vi "RT_Main.vi"() -> ()   [LabVIEW 2024]
uses:
  Type Definitions/FIFO_Health.ctl
  Type Definitions/FPGA_routine_pulsing_typedef.ctl
  <vilib>/Utility/error.llb/Error Cluster From Error Code.vi
  <vilib>/rvi/errors/niLvFpgaAdjustHostInterfaceError.vi
  <vilib>/RVI Host/nirviSupport.llb/nirviErrorClusterFromErrorCode.vi
  <vilib>/rvi/interface/nirviReadWriteControl/nirviReadWriteControl.xnode
  <vilib>/rvi/interface/nirviMethod/nirviMethod.xnode
  <vilib>/FPGAPlugInAG/Dynamic/niLvFpga_ReadFifo_Dynamic.vi
  <vilib>/rvi/errors/niLvFpgaMergeErrorWithErrorCode.vi
  NiFpgaLv.dll
  <vilib>/rvi/interface/Simulation/niFpgaSimulationCallBeginRW.vi
  <vilib>/rvi/interface/nirviMethod/StockFPGA_InlinedMethodWaitForMultipleIRQ.vi
  <vilib>/FPGAPlugInAG/Dynamic/niLvFpga_WaitOnIrq_Dynamic.vi
  <vilib>/FPGAPlugInAG/Dynamic/niLvFpga_AcknowledgeIrq_Dynamic.vi
  <vilib>/rvi/interface/nirviMethod/StockFPGA_InlinedMethodWaitForSingleIRQ.vi
panel:
  out "Data Streaming Start":bool
  out "Triggers Start":bool
  out "Packet Start":bool
  out "RT_FPGA_FIFO_health":T1
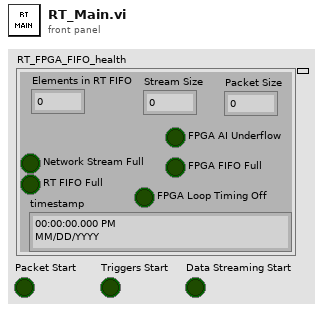
[diagram p1: front panel]
types:
  T1 = typedef "FIFO_Health.ctl" = cluster{"Elements in RT FIFO":i32, "Network Stream Full":bool, "RT FIFO Full":bool, "FPGA AI Underflow":bool, "FPGA FIFO Full":bool, "FPGA Loop Timing Off":bool, "timestamp":timestamp, "Stream Size":u32, "Packet Size":u32}
  T2 = cluster{"RT FIFO":refnum<k33>, "RT writer":refnum<k21>}
  T3 = typedef "FPGA_routine_pulsing_typedef.ctl" = cluster{"Pulsing":bool, "Pulse duration (uS)":u32, "Pulse Period (uS)":u32}
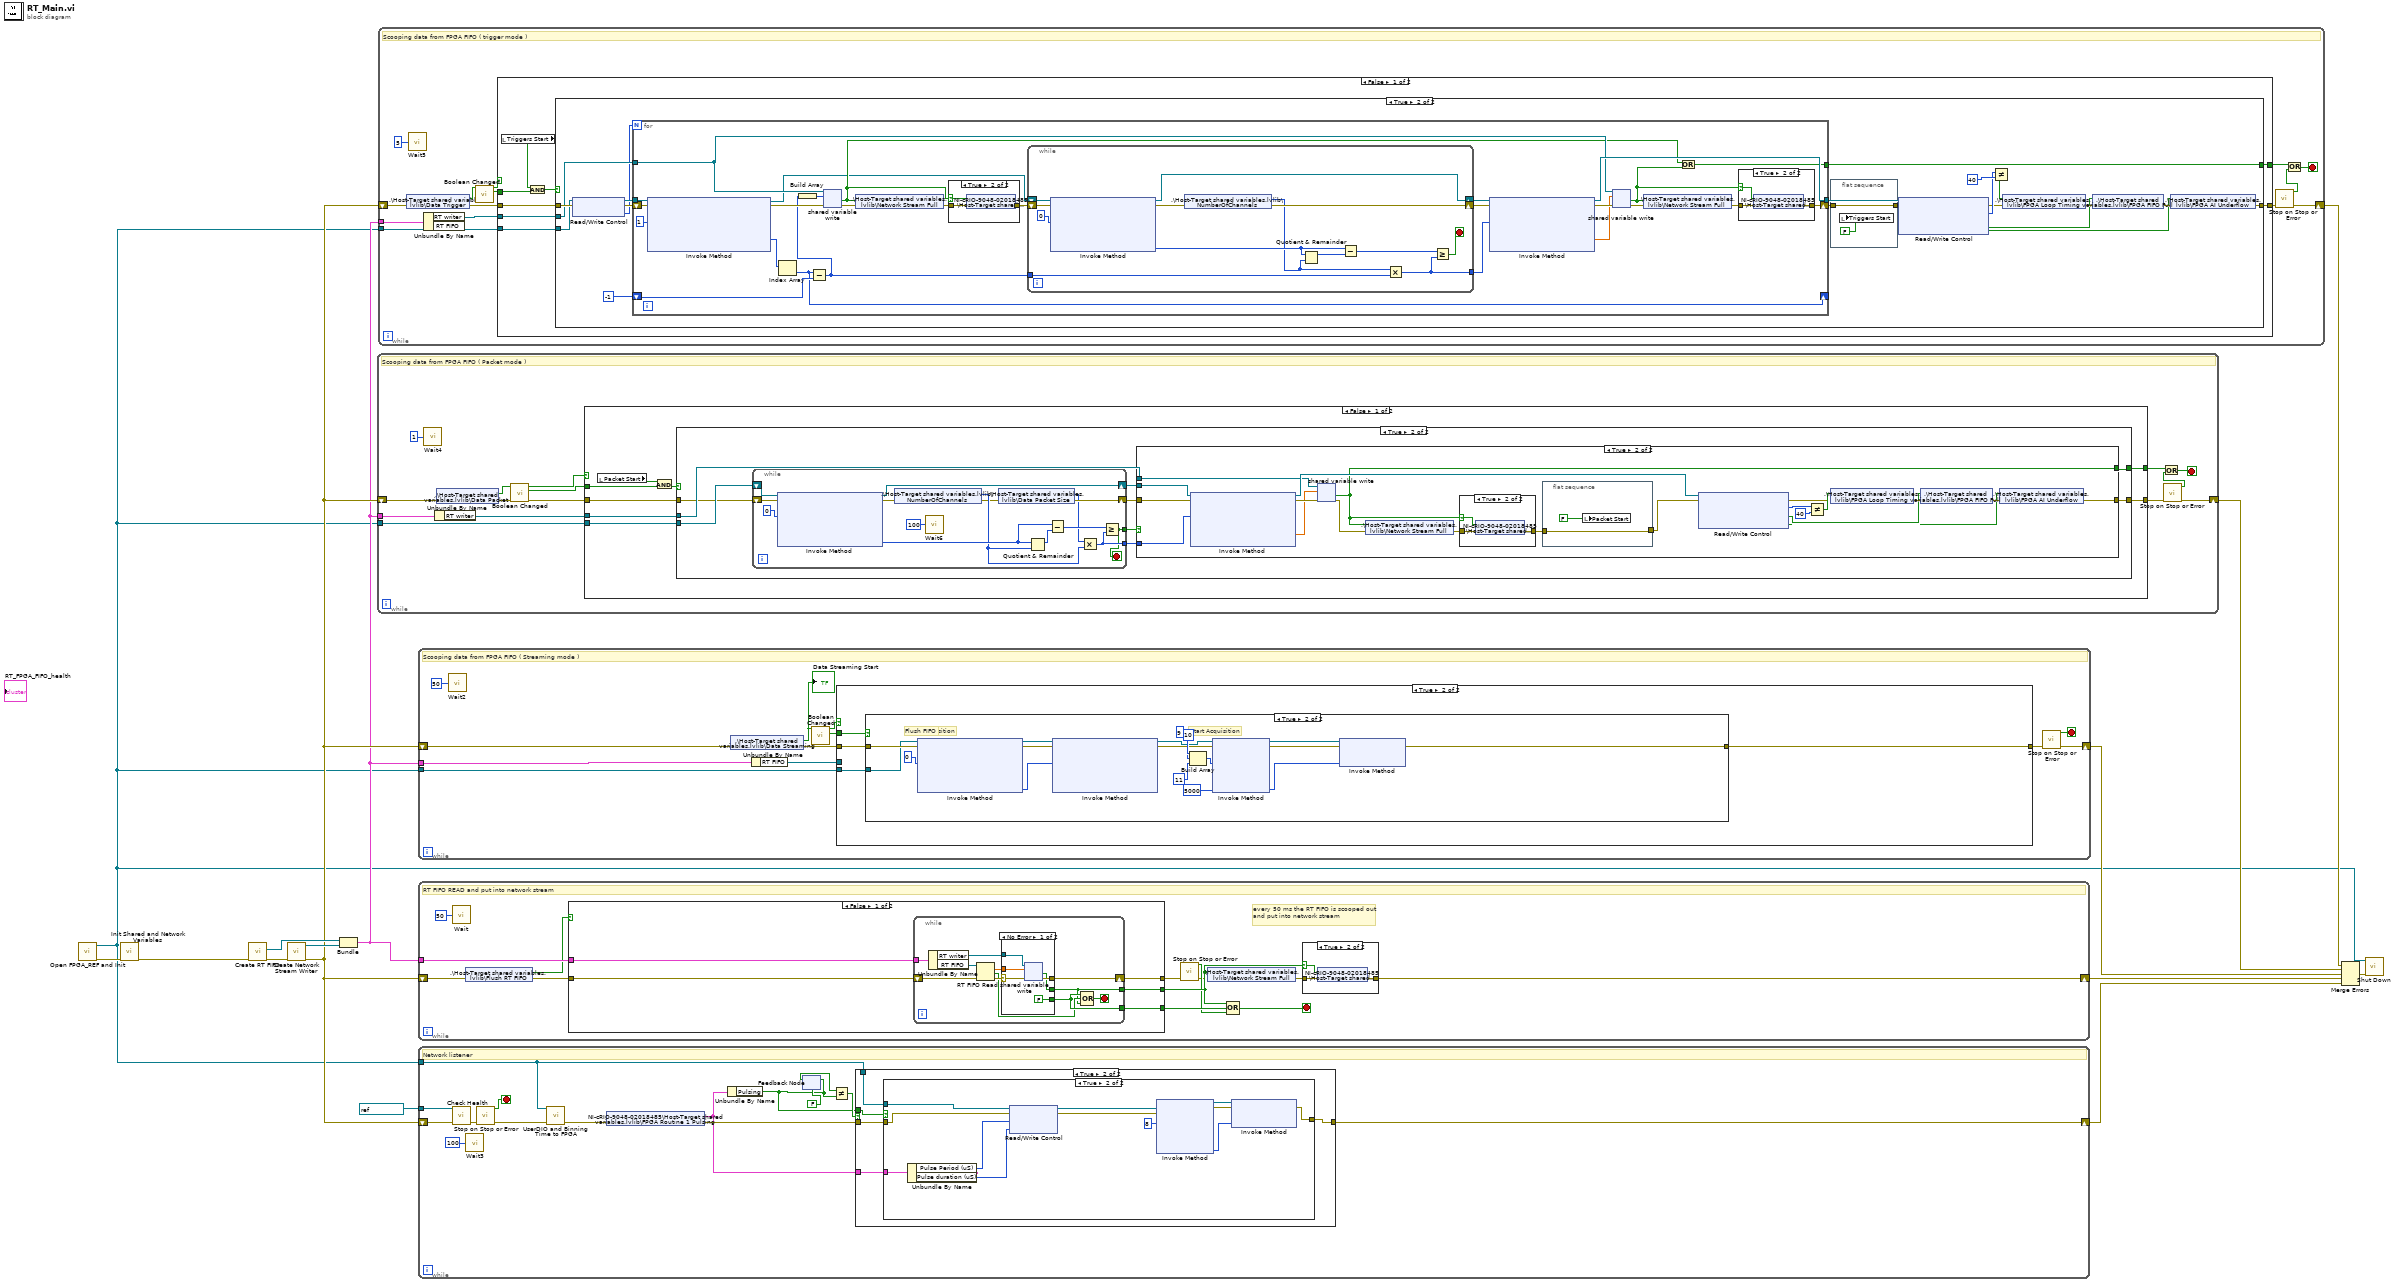
[diagram p0: block diagram]
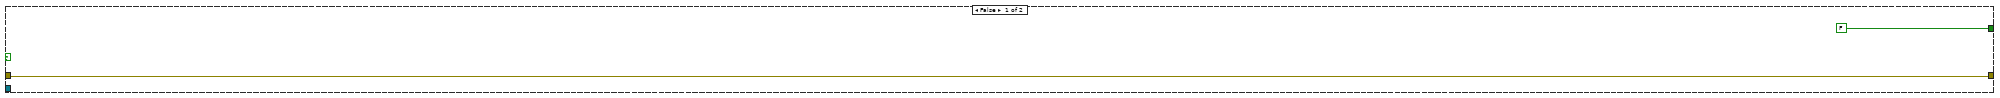
[diagram p2: hidden frame]
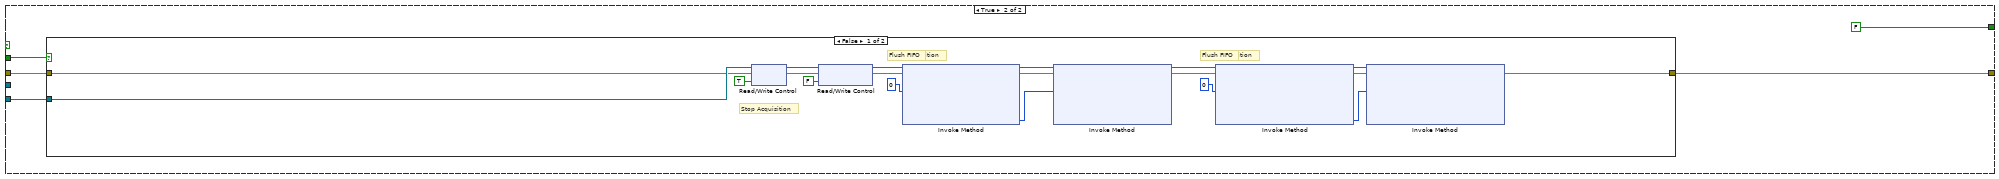
[diagram p5: hidden frame]
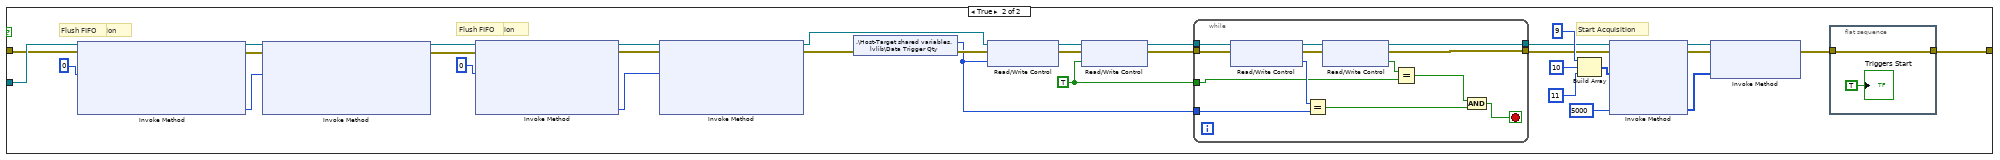
[diagram p6: hidden frame]
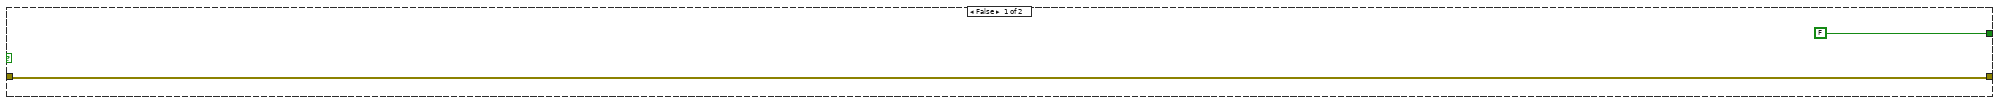
[diagram p7: hidden frame]
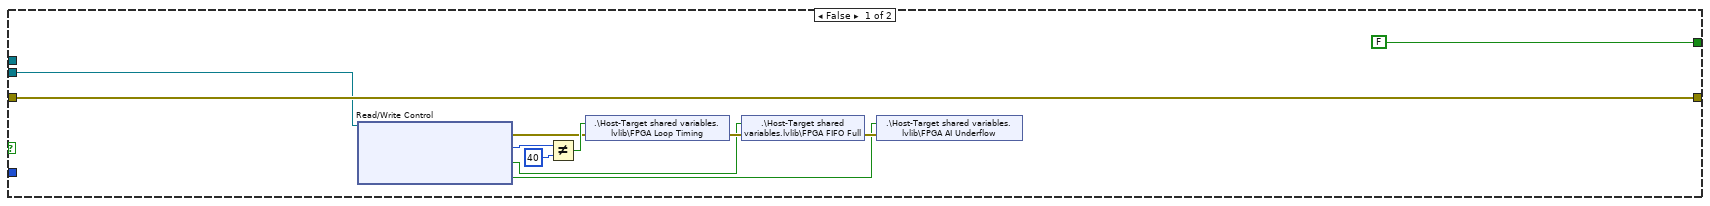
[diagram p8: hidden frame]
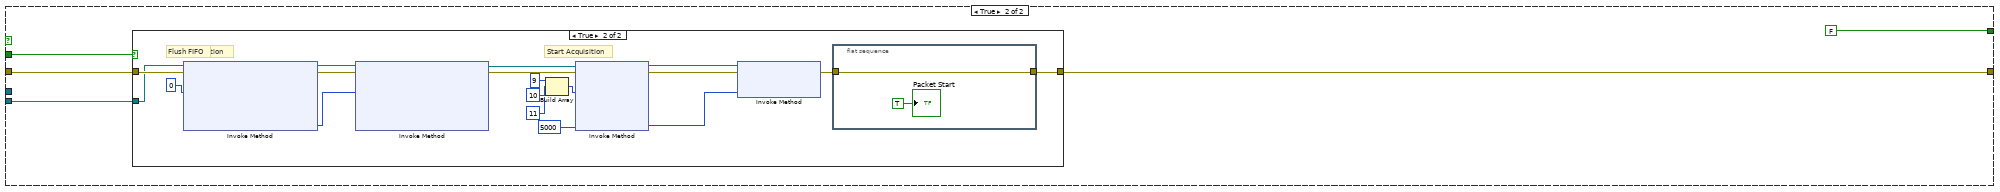
[diagram p10: hidden frame]
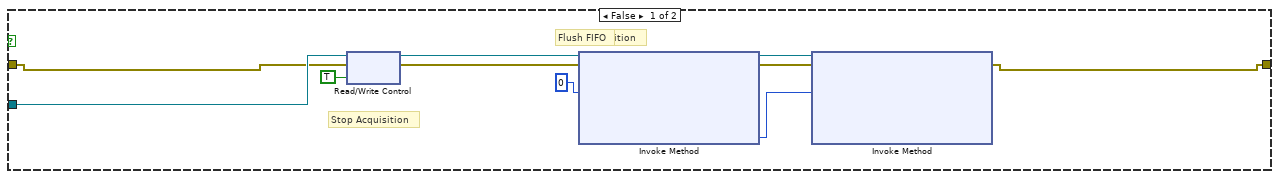
[diagram p11: hidden frame]
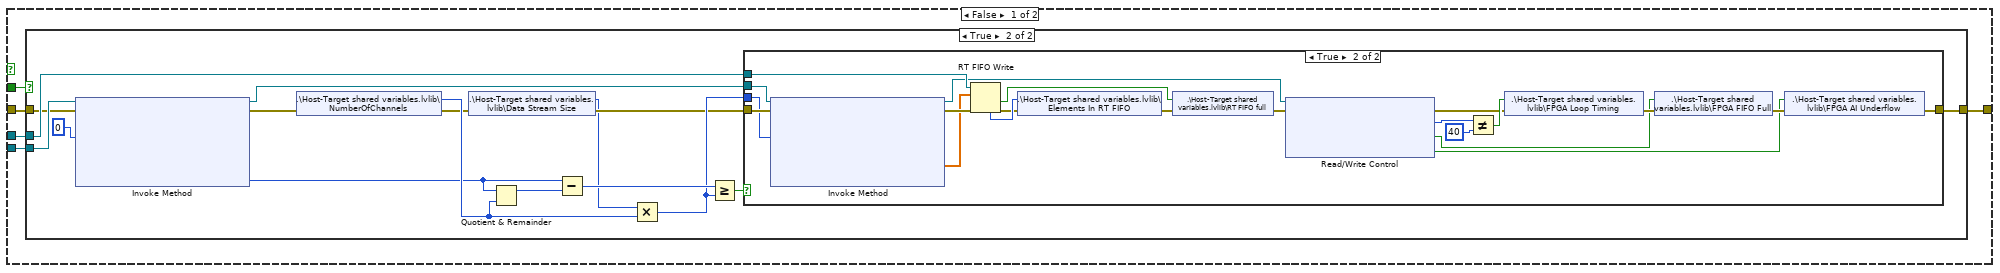
[diagram p12: hidden frame]
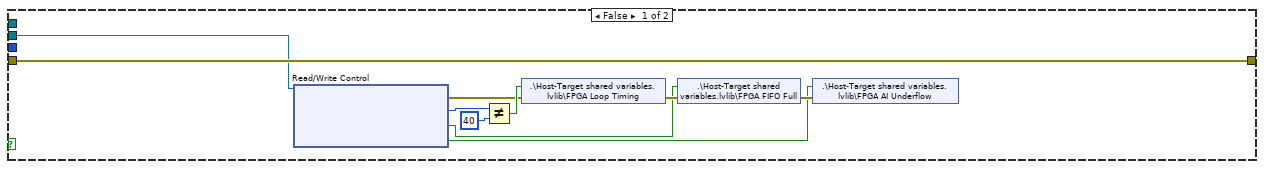
[diagram p14: hidden frame]
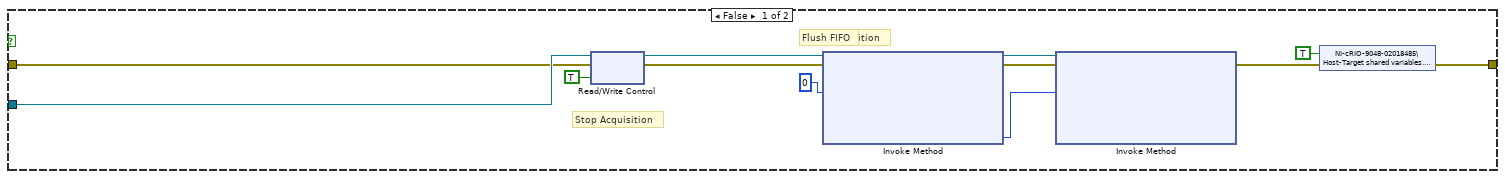
[diagram p15: hidden frame]
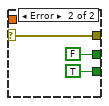
[diagram p16: hidden frame]
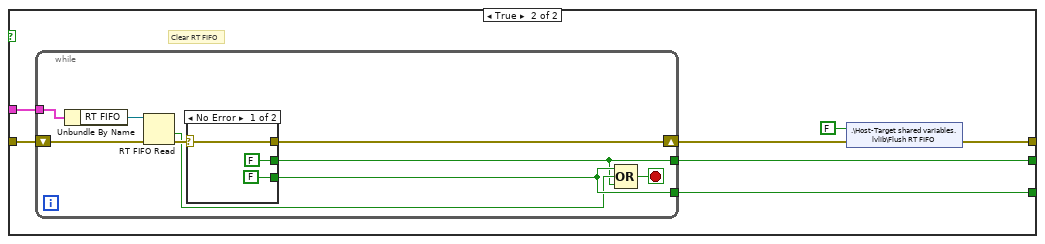
[diagram p17: hidden frame]
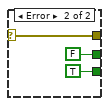
[diagram p18: hidden frame]
diagram:
  n1 = call "Open FPGA_REF and Init.vi"() -> ("error out"=w15:errorcluster, "FPGA VI Reference Out"=w1:refnum<k20>)  [unwired: 10 in]
  n2 = call "Init Shared and Network Variables.vi"("error in (no error)"=w15) -> ("error out"=w2:errorcluster)  [unwired: 10 in]
  n3 = call "Create RT FIFO.vi"("error in (no error)"=w2) -> ("error out"=w14:errorcluster, "RT FIFO"=w13:refnum<k33>)  [unwired: 9 in]
  n4 = call "Create Network Stream Writer.vi"("error in (no error)"=w14) -> ("error out"=w6:errorcluster, "RT writer"=w9:refnum<k21>)  [unwired: 9 in]
  n5 = Bundle("RT FIFO"=w13, "RT writer"=w9) -> (w5:T2)  [unwired: 1 in]
  n6 = while {
    shift-right: [w24] -> w8
    shift-left: w6 -> [w16]
    tunnel: w1 -> [w27]
    tunnel: w5 -> [w26]
    stop <- w20 stop-if-true
    # "Scooping data from FPGA FIFO ( Packet mode )"
    n7 = call "Wait4"("Count(mSec)"=u32 1) -> ()  [unwired: 1 out]
    n8 = Unbundle By Name(w26) -> ("RT writer"=w25:refnum<k21>)
    n9 = shared-variable ".\\Host-Target shared variables.lvlib\\Data Packet"(error in=w16) -> (w30:bool, error out=w18:errorcluster)
    n10 = call "Boolean Changed.vi"("error in (no error)"=w18, "Boolean in"=w30) -> ("error in (no error) 2"=w17:errorcluster, "Value"=w28:bool, "Changed?"=w29:bool)  [unwired: 6 in]
    n11 = case shown="False" w29 {
      tunnel: w17 -> [w37 w107]
      tunnel: [w36 w103] -> w23
      tunnel: w28 -> [w38 w106]
      tunnel: w27 -> [w35 w105]
      tunnel: w25 -> [w34 _]
      tunnel: [w33 FALSE] -> w19
      frame False {
        n12 = local read "Packet Start"() -> (w31:bool)
        n13 = And(x=w31, y=w38) -> (x .and. y?=w32:bool)
        n14 = case shown="True" w32 {
          tunnel: [w39 w46] -> w36
          tunnel: w37 -> [w39 w41]
          tunnel: w35 -> [_ w48]
          tunnel: w34 -> [_ w45]
          tunnel: [FALSE w42] -> w33
          frame False {
          }
          frame True {
            n15 = while {
              tunnel: [w51] -> w47
              tunnel: [w56] -> w44
              shift-right: [w63] -> w49
              shift-left: w48 -> [w60]
              shift-right: [w54] -> w43
              shift-left: w41 -> [w52]
              stop <- w51 stop-if-true
              n16 = xnode "Invoke Method"("FPGA VI Reference In"=w60, "error in"=w52, "Number of Elements"=u32 0) -> ("FPGA VI Reference Out"=w63:refnum<k20>, "error out"=w59:errorcluster, "Elements Remaining"=w61:u32)  [unwired: 1 in, 1 out]
              n17 = shared-variable ".\\Host-Target shared variables.lvlib\\NumberOfChannels"(error in=w59) -> (w57:u8, error out=w55:errorcluster)
              n18 = call "Wait6"("Count(uSec)"=u32 100) -> ()  [unwired: 1 out]
              n19 = shared-variable ".\\Host-Target shared variables.lvlib\\Data Packet Size"(error in=w55) -> (w53:u32, error out=w54:errorcluster)
              n20 = Quotient & Remainder(x=w61, y=w57) -> (x-y*floor(x/y)=w62:u32)  [unwired: 1 out]
              n21 = Subtract(x=w61, y=w62) -> (x-y=w58:u32)
              n22 = Multiply(x=w53, y=w57) -> (x*y=w56:u32)
              n23 = Greater Or Equal?(x=w58, y=w56) -> (x >= y?=w51:bool)
            }
            n24 = case shown="True" w47 {
              tunnel: w49 -> [w66 w96]
              tunnel: w43 -> [w75 w95]
              tunnel: w44 -> [_ w94]
              tunnel: [w75 w76] -> w46
              tunnel: w45 -> [_ w83]
              tunnel: [FALSE w79] -> w42
              frame False {
                n25 = xnode "Read/Write Control"("FPGA VI Reference In"=w66) -> ("error out"=w71:errorcluster, "Actual Loop Period (ticks)"=w73:u32, "DMA FIFO Full"=w68:bool, "Module Underflow"=w67:bool)  [unwired: 1 in, 1 out]
                n26 = Not Equal?(x=w73, y=u32 40) -> (x != y?=w72:bool)
                n27 = shared-variable ".\\Host-Target shared variables.lvlib\\FPGA Loop Timing"(w72, error in=w71) -> (error out=w70:errorcluster)
                n28 = shared-variable ".\\Host-Target shared variables.lvlib\\FPGA FIFO Full"(w68, error in=w70) -> (error out=w69:errorcluster)
                n29 = shared-variable ".\\Host-Target shared variables.lvlib\\FPGA AI Underflow"(w67, error in=w69) -> ()  [unwired: 1 out]
              }
              frame True {
                n30 = xnode "Invoke Method"("FPGA VI Reference In"=w96, "error in"=w95, "Number of Elements"=w94) -> ("FPGA VI Reference Out"=w93:refnum<k20>, "error out"=w84:errorcluster, "Data"=w80:sgl[])  [unwired: 1 in, 1 out]
                n31 = shared-variable-write(w83, w84, w80) -> (w81:errorcluster, w79:bool)  [unwired: 1 in, 1 out]
                n32 = shared-variable ".\\Host-Target shared variables.lvlib\\Network Stream Full"(w79, error in=w81) -> (error out=w82:errorcluster)
                n33 = case shown="True" w79 {
                  selector: w79 -> [_ w102]
                  tunnel: w82 -> [w99 w101]
                  tunnel: [w99 w100] -> w78
                  frame False {
                  }
                  frame True {
                    n34 = shared-variable "NI-cRIO-9048-02018485\\Host-Target shared variables.lvlib\\Stop RT"(w102, error in=w101) -> (error out=w100:errorcluster)
                  }
                }
                n35 = flat-sequence {
                  tunnel: w78 -> [w98]
                  tunnel: [w98] -> w77
                  frame #0 {
                    n36 = local write "Packet Start"(FALSE ("Data Packet")) -> ()
                  }
                }
                n37 = xnode "Read/Write Control"("FPGA VI Reference In"=w93, "error in"=w77) -> ("error out"=w89:errorcluster, "Actual Loop Period (ticks)"=w91:u32, "DMA FIFO Full"=w86:bool, "Module Underflow"=w85:bool)  [unwired: 1 out]
                n38 = Not Equal?(x=w91, y=u32 40) -> (x != y?=w90:bool)
                n39 = shared-variable ".\\Host-Target shared variables.lvlib\\FPGA Loop Timing"(w90, error in=w89) -> (error out=w88:errorcluster)
                n40 = shared-variable ".\\Host-Target shared variables.lvlib\\FPGA FIFO Full"(w86, error in=w88) -> (error out=w87:errorcluster)
                n41 = shared-variable ".\\Host-Target shared variables.lvlib\\FPGA AI Underflow"(w85, error in=w87) -> (error out=w76:errorcluster)
              }
            }
          }
        }
      }
      frame True {
        n42 = case shown="True" w106 {
          tunnel: w107 -> [w108 w121]
          tunnel: [w109 w126] -> w103
          tunnel: w105 -> [w113 w119]
          frame False {
            # "Flush FIFO"
            # "Stop Acquisition"
            # "Stop Acquisition"
            n43 = xnode "Read/Write Control"("FPGA VI Reference In"=w113, "error in"=w108, "Stop"=TRUE) -> ("FPGA VI Reference Out"=w111:refnum<k20>, "error out"=w110:errorcluster)
            n44 = xnode "Invoke Method"("FPGA VI Reference In"=w111, "error in"=w110, "Number of Elements"=u32 0) -> ("FPGA VI Reference Out"=w115:refnum<k20>, "error out"=w114:errorcluster, "Elements Remaining"=w116:u32)  [unwired: 1 in, 1 out]
            n45 = xnode "Invoke Method"("FPGA VI Reference In"=w115, "error in"=w114, "Number of Elements"=w116) -> ("error out"=w109:errorcluster)  [unwired: 1 in, 3 out]
          }
          frame True {
            # "Flush FIFO"
            # "Stop Acquisition"
            # "Start Acquisition"
            n46 = xnode "Invoke Method"("FPGA VI Reference In"=w119, "error in"=w121, "Number of Elements"=u32 0) -> ("FPGA VI Reference Out"=w124:refnum<k20>, "error out"=w125:errorcluster, "Elements Remaining"=w123:u32)  [unwired: 1 in, 1 out]
            n47 = xnode "Invoke Method"("FPGA VI Reference In"=w124, "error in"=w125, "Number of Elements"=w123) -> ("FPGA VI Reference Out"=w118:refnum<k20>, "error out"=w120:errorcluster)  [unwired: 1 in, 2 out]
            n48 = Build Array(9 ("element"), 10 ("element"), 11 ("element")) -> (w128:i32[])
            n49 = xnode "Invoke Method"("FPGA VI Reference In"=w118, "error in"=w120, "IRQ Number(s)"=w128, "Timeout (ms)"=5000) -> ("FPGA VI Reference Out"=w135:refnum<k20>, "error out"=w134:errorcluster, "IRQ(s) Asserted"=w133:i32[])  [unwired: 1 out]
            n50 = xnode "Invoke Method"("FPGA VI Reference In"=w135, "error in"=w134, "IRQ Number(s)"=w133) -> ("error out"=w127:errorcluster)  [unwired: 1 out]
            n51 = flat-sequence {
              tunnel: w127 -> [w137]
              tunnel: [w137] -> w126
              frame #0 {
                "Packet Start" <- TRUE ("Packet Start")
              }
            }
          }
        }
      }
    }
    n52 = call "Stop on Stop or Error.vi"("error in (no error)"=w23) -> ("error out"=w24:errorcluster, "Boolean"=w21:bool)  [unwired: 9 in]
    n53 = Or(x=w19, y=w21) -> (x .or. y?=w20:bool)
  }
  n54 = while {
    shift-right: [w145] -> w4
    shift-left: w6 -> [w151]
    tunnel: w1 -> [w146]
    tunnel: w5 -> [w142]
    stop <- w138 stop-if-true
    # "Scooping data from FPGA FIFO ( trigger mode )"
    n55 = shared-variable ".\\Host-Target shared variables.lvlib\\Data Trigger"(error in=w151) -> (w150:bool, error out=w148:errorcluster)
    n56 = call "Wait5"("Count(mSec)"=u32 5) -> ()  [unwired: 1 out]
    n57 = Unbundle By Name(w142) -> ("RT writer"=w141:refnum<k21>)  [unwired: 1 out]
    n58 = call "Boolean Changed.vi"("Boolean in"=w150) -> ("Value"=w147:bool, "Changed?"=w149:bool)  [unwired: 7 in, 1 out]
    n59 = case shown="False" w149 {
      tunnel: w148 -> [w159 w235]
      tunnel: [w158 w234] -> w144
      tunnel: w147 -> [w153 w233]
      tunnel: w146 -> [w157 w232]
      tunnel: w141 -> [w156 _]
      tunnel: [w155 FALSE] -> w140
      frame False {
        n60 = local read "Triggers Start"() -> (w152:bool)
        n61 = And(x=w152, y=w153) -> (x .and. y?=w154:bool)
        n62 = case shown="True" w154 {
          tunnel: [w161 w181] -> w158
          tunnel: w159 -> [w161 w180]
          tunnel: w157 -> [_ w166]
          tunnel: w156 -> [_ w167]
          tunnel: [FALSE w168] -> w155
          frame False {
          }
          frame True {
            n63 = xnode "Read/Write Control"("FPGA VI Reference In"=w166, "error in"=w180) -> ("FPGA VI Reference Out"=w178:refnum<k20>, "error out"=w179:errorcluster, "Total Triggers"=w165:u32)
            n64 = for {
              N: w165 -> [_]
              shift-right: [w202] -> w163
              shift-left: w179 -> [w193]
              tunnel: w178 -> [w189]
              tunnel: [w206] -> w177
              tunnel: [w195] -> w168
              tunnel: w167 -> [w200]
              shift-right: [w186] -> _
              shift-left: -1 -> [w187]
              n65 = xnode "Invoke Method"("FPGA VI Reference In"=w189, "error in"=w193, "Number of Elements"=u32 1) -> ("FPGA VI Reference Out"=w188:refnum<k20>, "error out"=w192:errorcluster, "Data"=w190:u32[])  [unwired: 1 in, 1 out]
              n66 = Index Array(array=w190) -> (element=w186:u32)  [unwired: 1 in]
              n67 = Subtract(x=w186, y=w187) -> (x-y=w185:u32)
              n68 = Build Array(w185) -> (w184:u32[])
              n69 = shared-variable-write(w200, w192, w184) -> (w198:errorcluster, w196:bool)  [unwired: 1 in, 1 out]
              n70 = shared-variable ".\\Host-Target shared variables.lvlib\\Network Stream Full"(w196, error in=w198) -> (error out=w199:errorcluster)
              n71 = case shown="True" w196 {
                selector: w196 -> [_ w213]
                tunnel: w199 -> [w210 w212]
                tunnel: [w210 w211] -> w194
                frame False {
                }
                frame True {
                  n72 = shared-variable "NI-cRIO-9048-02018485\\Host-Target shared variables.lvlib\\Stop RT"(w213, error in=w212) -> (error out=w211:errorcluster)
                }
              }
              n73 = while {
                tunnel: [w220] -> w208
                shift-right: [w225] -> w209
                shift-left: w188 -> [w218]
                shift-right: [w219] -> w207
                shift-left: w194 -> [w217]
                tunnel: w185 -> [w214]
                stop <- w216 stop-if-true
                n74 = xnode "Invoke Method"("FPGA VI Reference In"=w218, "error in"=w217, "Number of Elements"=u32 0) -> ("FPGA VI Reference Out"=w225:refnum<k20>, "error out"=w222:errorcluster, "Elements Remaining"=w223:u32)  [unwired: 1 in, 1 out]
                n75 = shared-variable ".\\Host-Target shared variables.lvlib\\NumberOfChannels"(error in=w222) -> (w215:u8, error out=w219:errorcluster)
                n76 = Quotient & Remainder(x=w223, y=w215) -> (x-y*floor(x/y)=w224:u32)  [unwired: 1 out]
                n77 = Subtract(x=w223, y=w224) -> (x-y=w221:u32)
                n78 = Multiply(x=w215, y=w214) -> (x*y=w220:u32)
                n79 = Greater Or Equal?(x=w221, y=w220) -> (x >= y?=w216:bool)
              }
              n80 = xnode "Invoke Method"("FPGA VI Reference In"=w209, "error in"=w207, "Number of Elements"=w208) -> ("FPGA VI Reference Out"=w206:refnum<k20>, "error out"=w205:errorcluster, "Data"=w201:sgl[])  [unwired: 1 in, 1 out]
              n81 = shared-variable-write(w200, w205, w201) -> (w204:errorcluster, w197:bool)  [unwired: 1 in, 1 out]
              n82 = shared-variable ".\\Host-Target shared variables.lvlib\\Network Stream Full"(w197, error in=w204) -> (error out=w203:errorcluster)
              n83 = Or(x=w196, y=w197) -> (x .or. y?=w195:bool)
              n84 = case shown="True" w197 {
                selector: w197 -> [_ w230]
                tunnel: w203 -> [w227 w229]
                tunnel: [w227 w228] -> w202
                frame False {
                }
                frame True {
                  n85 = shared-variable "NI-cRIO-9048-02018485\\Host-Target shared variables.lvlib\\Stop RT"(w230, error in=w229) -> (error out=w228:errorcluster)
                }
              }
            }
            n86 = flat-sequence {
              tunnel: w163 -> [w183]
              tunnel: [w183] -> w162
              frame #0 {
                n87 = local write "Triggers Start"(FALSE ("Triggers Start")) -> ()
              }
            }
            n88 = xnode "Read/Write Control"("FPGA VI Reference In"=w177, "error in"=w162) -> ("error out"=w173:errorcluster, "Actual Loop Period (ticks)"=w175:u32, "DMA FIFO Full"=w170:bool, "Module Underflow"=w169:bool)  [unwired: 1 out]
            n89 = Not Equal?(x=w175, y=u32 40) -> (x != y?=w174:bool)
            n90 = shared-variable ".\\Host-Target shared variables.lvlib\\FPGA Loop Timing"(w174, error in=w173) -> (error out=w172:errorcluster)
            n91 = shared-variable ".\\Host-Target shared variables.lvlib\\FPGA FIFO Full"(w170, error in=w172) -> (error out=w171:errorcluster)
            n92 = shared-variable ".\\Host-Target shared variables.lvlib\\FPGA AI Underflow"(w169, error in=w171) -> (error out=w181:errorcluster)
          }
        }
      }
      frame True {
        n93 = case shown="False" w233 {
          tunnel: w235 -> [w249 w266]
          tunnel: [w242 w263] -> w234
          tunnel: w232 -> [w250 w268]
          frame False {
            # "Flush FIFO"
            # "Stop Acquisition"
            # "Flush FIFO"
            # "Stop Acquisition"
            # "Stop Acquisition"
            n94 = xnode "Read/Write Control"("FPGA VI Reference In"=w250, "error in"=w249, "Stop"=TRUE) -> ("FPGA VI Reference Out"=w238:refnum<k20>, "error out"=w240:errorcluster)
            n95 = xnode "Read/Write Control"("FPGA VI Reference In"=w238, "error in"=w240, "Use Triggers"=FALSE) -> ("FPGA VI Reference Out"=w237:refnum<k20>, "error out"=w239:errorcluster)
            n96 = xnode "Invoke Method"("FPGA VI Reference In"=w237, "error in"=w239, "Number of Elements"=u32 0) -> ("FPGA VI Reference Out"=w252:refnum<k20>, "error out"=w251:errorcluster, "Elements Remaining"=w253:u32)  [unwired: 1 in, 1 out]
            n97 = xnode "Invoke Method"("FPGA VI Reference In"=w252, "error in"=w251, "Number of Elements"=w253) -> ("FPGA VI Reference Out"=w241:refnum<k20>, "error out"=w243:errorcluster)  [unwired: 1 in, 2 out]
            n98 = xnode "Invoke Method"("FPGA VI Reference In"=w241, "error in"=w243, "Number of Elements"=u32 0) -> ("FPGA VI Reference Out"=w245:refnum<k20>, "error out"=w244:errorcluster, "Elements Remaining"=w246:u32)  [unwired: 1 in, 1 out]
            n99 = xnode "Invoke Method"("FPGA VI Reference In"=w245, "error in"=w244, "Number of Elements"=w246) -> ("error out"=w242:errorcluster)  [unwired: 1 in, 3 out]
          }
          frame True {
            w255 = TRUE ("Use Triggers")
            # "Flush FIFO"
            # "Stop Acquisition"
            # "Flush FIFO"
            # "Stop Acquisition"
            # "Start Acquisition"
            n100 = xnode "Invoke Method"("FPGA VI Reference In"=w268, "error in"=w266, "Number of Elements"=u32 0) -> ("FPGA VI Reference Out"=w271:refnum<k20>, "error out"=w272:errorcluster, "Elements Remaining"=w270:u32)  [unwired: 1 in, 1 out]
            n101 = xnode "Invoke Method"("FPGA VI Reference In"=w271, "error in"=w272, "Number of Elements"=w270) -> ("FPGA VI Reference Out"=w267:refnum<k20>, "error out"=w265:errorcluster)  [unwired: 1 in, 2 out]
            n102 = xnode "Invoke Method"("FPGA VI Reference In"=w267, "error in"=w265, "Number of Elements"=u32 0) -> ("FPGA VI Reference Out"=w278:refnum<k20>, "error out"=w279:errorcluster, "Elements Remaining"=w277:u32)  [unwired: 1 in, 1 out]
            n103 = xnode "Invoke Method"("FPGA VI Reference In"=w278, "error in"=w279, "Number of Elements"=w277) -> ("FPGA VI Reference Out"=w274:refnum<k20>, "error out"=w275:errorcluster)  [unwired: 1 in, 2 out]
            n104 = shared-variable ".\\Host-Target shared variables.lvlib\\Data Trigger Qty"(error in=w275) -> (w256:u32, error out=w273:errorcluster)
            n105 = xnode "Read/Write Control"("FPGA VI Reference In"=w274, "error in"=w273, "Total Triggers"=w256) -> ("FPGA VI Reference Out"=w261:refnum<k20>, "error out"=w262:errorcluster)
            n106 = xnode "Read/Write Control"("FPGA VI Reference In"=w261, "error in"=w262, "Use Triggers"=w255) -> ("FPGA VI Reference Out"=w258:refnum<k20>, "error out"=w260:errorcluster)
            n107 = while {
              tunnel: w260 -> [w300]
              tunnel: [w298] -> w259
              tunnel: w258 -> [w297]
              tunnel: [w295] -> w257
              tunnel: w256 -> [w292]
              tunnel: w255 -> [w289]
              stop <- w294 stop-if-true
              n108 = xnode "Read/Write Control"("FPGA VI Reference In"=w297, "error in"=w300) -> ("FPGA VI Reference Out"=w296:refnum<k20>, "error out"=w299:errorcluster, "Total Triggers"=w293:u32)
              n109 = Equal?(x=w293, y=w292) -> (x = y?=w291:bool)
              n110 = xnode "Read/Write Control"("FPGA VI Reference In"=w296, "error in"=w299) -> ("FPGA VI Reference Out"=w295:refnum<k20>, "error out"=w298:errorcluster, "Use Triggers"=w290:bool)
              n111 = Equal?(x=w290, y=w289) -> (x = y?=w288:bool)
              n112 = And(x=w288, y=w291) -> (x .and. y?=w294:bool)
            }
            n113 = Build Array(9 ("element"), 10 ("element"), 11 ("element")) -> (w280:i32[])
            n114 = xnode "Invoke Method"("FPGA VI Reference In"=w257, "error in"=w259, "IRQ Number(s)"=w280, "Timeout (ms)"=5000) -> ("FPGA VI Reference Out"=w287:refnum<k20>, "error out"=w286:errorcluster, "IRQ(s) Asserted"=w285:i32[])  [unwired: 1 out]
            n115 = xnode "Invoke Method"("FPGA VI Reference In"=w287, "error in"=w286, "IRQ Number(s)"=w285) -> ("error out"=w264:errorcluster)  [unwired: 1 out]
            n116 = flat-sequence {
              tunnel: w264 -> [w302]
              tunnel: [w302] -> w263
              frame #0 {
                "Triggers Start" <- TRUE ("Triggers Start")
              }
            }
          }
        }
      }
    }
    n117 = call "Stop on Stop or Error.vi"("error in (no error)"=w144) -> ("error out"=w145:errorcluster, "Boolean"=w139:bool)  [unwired: 9 in]
    n118 = Or(x=w140, y=w139) -> (x .or. y?=w138:bool)
  }
  n119 = while {
    shift-right: [w306] -> w12
    shift-left: w6 -> [w314]
    tunnel: w1 -> [w309]
    tunnel: w5 -> [w308]
    stop <- w304 stop-if-true
    # "Scooping data from FPGA FIFO ( Streaming mode )"
    n120 = call "Wait2"("Count(mSec)"=u32 50) -> ()  [unwired: 1 out]
    n121 = shared-variable ".\\Host-Target shared variables.lvlib\\Data Streaming"(error in=w314) -> (w313:bool, error out=w311:errorcluster)
    "Data Streaming Start" <- w313
    n122 = Unbundle By Name(w308) -> ("RT FIFO"=w307:refnum<k33>)
    n123 = call "Boolean Changed.vi"("Boolean in"=w313) -> ("Value"=w310:bool, "Changed?"=w312:bool)  [unwired: 7 in, 1 out]
    n124 = case shown="True" w312 {
      tunnel: w311 -> [w318 w371]
      tunnel: [w317 w370] -> w305
      tunnel: w310 -> [w319 w369]
      tunnel: w309 -> [w316 w368]
      tunnel: w307 -> [w315 _]
      frame False {
        n125 = case shown="True" w319 {
          tunnel: [w320 w328] -> w317
          tunnel: w318 -> [w320 w321]
          tunnel: w316 -> [_ w333]
          tunnel: w315 -> [_ w327]
          frame False {
          }
          frame True {
            n126 = xnode "Invoke Method"("FPGA VI Reference In"=w333, "error in"=w321, "Number of Elements"=u32 0) -> ("FPGA VI Reference Out"=w335:refnum<k20>, "error out"=w332:errorcluster, "Elements Remaining"=w322:u32)  [unwired: 1 in, 1 out]
            n127 = shared-variable ".\\Host-Target shared variables.lvlib\\NumberOfChannels"(error in=w332) -> (w329:u8, error out=w325:errorcluster)
            n128 = shared-variable ".\\Host-Target shared variables.lvlib\\Data Stream Size"(error in=w325) -> (w323:u32, error out=w324:errorcluster)
            n129 = Quotient & Remainder(x=w322, y=w329) -> (x-y*floor(x/y)=w334:u32)  [unwired: 1 out]
            n130 = Subtract(x=w322, y=w334) -> (x-y=w331:u32)
            n131 = Multiply(x=w323, y=w329) -> (x*y=w326:u32)
            n132 = Greater Or Equal?(x=w331, y=w326) -> (x >= y?=w330:bool)
            n133 = case shown="True" w330 {
              tunnel: w335 -> [w337 w367]
              tunnel: w324 -> [w346 w366]
              tunnel: w326 -> [_ w365]
              tunnel: [w346 w351] -> w328
              tunnel: w327 -> [_ w363]
              frame False {
                n134 = xnode "Read/Write Control"("FPGA VI Reference In"=w337) -> ("error out"=w342:errorcluster, "Actual Loop Period (ticks)"=w344:u32, "DMA FIFO Full"=w339:bool, "Module Underflow"=w338:bool)  [unwired: 1 in, 1 out]
                n135 = Not Equal?(x=w344, y=u32 40) -> (x != y?=w343:bool)
                n136 = shared-variable ".\\Host-Target shared variables.lvlib\\FPGA Loop Timing"(w343, error in=w342) -> (error out=w341:errorcluster)
                n137 = shared-variable ".\\Host-Target shared variables.lvlib\\FPGA FIFO Full"(w339, error in=w341) -> (error out=w340:errorcluster)
                n138 = shared-variable ".\\Host-Target shared variables.lvlib\\FPGA AI Underflow"(w338, error in=w340) -> ()  [unwired: 1 out]
              }
              frame True {
                n139 = xnode "Invoke Method"("FPGA VI Reference In"=w367, "error in"=w366, "Number of Elements"=w365) -> ("FPGA VI Reference Out"=w357:refnum<k20>, "error out"=w364:errorcluster, "Data"=w362:sgl[])  [unwired: 1 in, 1 out]
                n140 = RT FIFO Write(0:w363, 1:w362, 3:w364) -> (7:w360:u32, 10:w361:bool, 11:w359:errorcluster)  [unwired: 2 in, 1 out]
                n141 = shared-variable ".\\Host-Target shared variables.lvlib\\Elements In RT FIFO"(w360, error in=w359) -> (error out=w358:errorcluster)
                n142 = shared-variable ".\\Host-Target shared variables.lvlib\\RT FIFO full"(w361, error in=w358) -> (error out=w356:errorcluster)
                n143 = xnode "Read/Write Control"("FPGA VI Reference In"=w357, "error in"=w356) -> ("error out"=w352:errorcluster, "Actual Loop Period (ticks)"=w354:u32, "DMA FIFO Full"=w348:bool, "Module Underflow"=w347:bool)  [unwired: 1 out]
                n144 = Not Equal?(x=w354, y=u32 40) -> (x != y?=w353:bool)
                n145 = shared-variable ".\\Host-Target shared variables.lvlib\\FPGA Loop Timing"(w353, error in=w352) -> (error out=w350:errorcluster)
                n146 = shared-variable ".\\Host-Target shared variables.lvlib\\FPGA FIFO Full"(w348, error in=w350) -> (error out=w349:errorcluster)
                n147 = shared-variable ".\\Host-Target shared variables.lvlib\\FPGA AI Underflow"(w347, error in=w349) -> (error out=w351:errorcluster)
              }
            }
          }
        }
      }
      frame True {
        n148 = case shown="True" w369 {
          tunnel: w371 -> [w378 w387]
          tunnel: [w373 w397] -> w370
          tunnel: w368 -> [w379 w385]
          frame False {
            # "Flush FIFO"
            # "Stop Acquisition"
            # "Stop Acquisition"
            n149 = xnode "Read/Write Control"("FPGA VI Reference In"=w379, "error in"=w378, "Stop"=TRUE) -> ("FPGA VI Reference Out"=w376:refnum<k20>, "error out"=w375:errorcluster)
            n150 = xnode "Invoke Method"("FPGA VI Reference In"=w376, "error in"=w375, "Number of Elements"=u32 0) -> ("FPGA VI Reference Out"=w381:refnum<k20>, "error out"=w380:errorcluster, "Elements Remaining"=w382:u32)  [unwired: 1 in, 1 out]
            n151 = xnode "Invoke Method"("FPGA VI Reference In"=w381, "error in"=w380, "Number of Elements"=w382) -> ("error out"=w374:errorcluster)  [unwired: 1 in, 3 out]
            n152 = shared-variable "NI-cRIO-9048-02018485\\Host-Target shared variables.lvlib\\Flush RT FIFO"(TRUE ("Flush RT FIFO"), error in=w374) -> (error out=w373:errorcluster)
          }
          frame True {
            # "Flush FIFO"
            # "Stop Acquisition"
            # "Start Acquisition"
            n153 = xnode "Invoke Method"("FPGA VI Reference In"=w385, "error in"=w387, "Number of Elements"=u32 0) -> ("FPGA VI Reference Out"=w390:refnum<k20>, "error out"=w391:errorcluster, "Elements Remaining"=w389:u32)  [unwired: 1 in, 1 out]
            n154 = xnode "Invoke Method"("FPGA VI Reference In"=w390, "error in"=w391, "Number of Elements"=w389) -> ("FPGA VI Reference Out"=w384:refnum<k20>, "error out"=w386:errorcluster)  [unwired: 1 in, 2 out]
            n155 = Build Array(9 ("element"), 10 ("element"), 11 ("element")) -> (w392:i32[])
            n156 = xnode "Invoke Method"("FPGA VI Reference In"=w384, "error in"=w386, "IRQ Number(s)"=w392, "Timeout (ms)"=5000) -> ("FPGA VI Reference Out"=w400:refnum<k20>, "error out"=w399:errorcluster, "IRQ(s) Asserted"=w398:i32[])  [unwired: 1 out]
            n157 = xnode "Invoke Method"("FPGA VI Reference In"=w400, "error in"=w399, "IRQ Number(s)"=w398) -> ("error out"=w397:errorcluster)  [unwired: 1 out]
          }
        }
      }
    }
    n158 = call "Stop on Stop or Error.vi"("error in (no error)"=w305) -> ("error out"=w306:errorcluster, "Boolean"=w304:bool)  [unwired: 9 in]
  }
  n159 = while {
    shift-right: [w408] -> w11
    shift-left: w6 -> [w403]
    tunnel: w5 -> [w412]
    stop <- w413 stop-if-true
    # "every 50 ms the RT FIFO is scooped out and put into network stream"
    # "RT FIFO READ and put into network stream"
    n160 = call "Wait"("Count(mSec)"=u32 50) -> ()  [unwired: 1 out]
    n161 = shared-variable ".\\Host-Target shared variables.lvlib\\Flush RT FIFO"(error in=w403) -> (w401:bool, error out=w402:errorcluster)
    n162 = case shown="False" w401 {
      tunnel: w412 -> [w418 w442]
      tunnel: w402 -> [w417 w445]
      tunnel: [w416 w443] -> w411
      tunnel: [w415 w444] -> w410
      tunnel: [w414 w441] -> w406
      frame False {
        n163 = while {
          tunnel: [w429] -> w416
          shift-right: [w423] -> w414
          shift-left: w417 -> [w424]
          tunnel: [w419] -> w415
          tunnel: w418 -> [w422]
          stop <- w425 stop-if-true
          n164 = Unbundle By Name(w422) -> ("RT writer"=w421:refnum<k21>, "RT FIFO"=w420:refnum<k33>)
          n165 = RT FIFO Read(0:w420, 3:w424) -> (9:w427:sgl[], 10:w426:bool, 11:w428:errorcluster)  [unwired: 2 in, 2 out]
          n166 = case shown="No Error" w428 {
            selector: w428 -> [w434 w437]
            tunnel: w427 -> [w430 _]
            tunnel: [FALSE ("value") TRUE ("value")] -> w429
            tunnel: [w433 w437] -> w423
            tunnel: [w432 FALSE] -> w419
            tunnel: w421 -> [w431 _]
            frame No Error {
              n167 = shared-variable-write(w431, w434, w430) -> (w433:errorcluster, w432:bool)  [unwired: 1 in, 1 out]
            }
            frame Error {
            }
          }
          n168 = Compound Arithmetic op=OR(w429, w426, w419) -> (w425:bool)
        }
      }
      frame True {
        # "Clear RT FIFO"
        n169 = while {
          tunnel: [w454] -> w443
          shift-right: [w449] -> w439
          shift-left: w445 -> [w450]
          tunnel: [w446] -> w444
          tunnel: w442 -> [w448]
          stop <- w451 stop-if-true
          n170 = Unbundle By Name(w448) -> ("RT FIFO"=w447:refnum<k33>)
          n171 = RT FIFO Read(0:w447, 3:w450) -> (10:w452:bool, 11:w453:errorcluster)  [unwired: 2 in, 3 out]
          n172 = case shown="No Error" w453 {
            selector: w453 -> [w456 w459]
            tunnel: [FALSE ("value") TRUE ("value")] -> w454
            tunnel: [w456 w459] -> w449
            tunnel: [FALSE FALSE] -> w446
            frame No Error {
            }
            frame Error {
            }
          }
          n173 = Compound Arithmetic op=OR(w454, w452, w446) -> (w451:bool)
        }
        n174 = shared-variable ".\\Host-Target shared variables.lvlib\\Flush RT FIFO"(FALSE ("Flush Network Stream"), error in=w439) -> (error out=w441:errorcluster)
      }
    }
    n175 = call "Stop on Stop or Error.vi"("error in (no error)"=w406) -> ("error out"=w405:errorcluster, "Boolean"=w407:bool)  [unwired: 9 in]
    n176 = shared-variable ".\\Host-Target shared variables.lvlib\\Network Stream Full"(w410, error in=w405) -> (error out=w409:errorcluster)
    n177 = Compound Arithmetic op=OR(w410, w411, w407) -> (w413:bool)
    n178 = case shown="True" w410 {
      selector: w410 -> [_ w464]
      tunnel: w409 -> [w461 w463]
      tunnel: [w461 w462] -> w408
      frame False {
      }
      frame True {
        n179 = shared-variable "NI-cRIO-9048-02018485\\Host-Target shared variables.lvlib\\Stop RT"(w464, error in=w463) -> (error out=w462:errorcluster)
      }
    }
  }
  n180 = while {
    shift-right: [w471] -> w3
    shift-left: w6 -> [w479]
    tunnel: w1 -> [w465]
    tunnel: refnum<k21> "localhost" ("System Session") -> [w468]
    stop <- w477 stop-if-true
    # "Network listener"
    n181 = call "Check Health.vi"("error in"=w479, "System Session"=w468) -> ("error out"=w478:errorcluster)  [unwired: 8 in, 1 out]
    n182 = call "Wait3"("Count(mSec)"=u32 100) -> ()  [unwired: 1 out]
    n183 = call "Stop on Stop or Error.vi"("error in (no error)"=w478) -> ("error out"=w467:errorcluster, "Boolean"=w477:bool)  [unwired: 9 in]
    n184 = call "UserDIO and Binning Time to FPGA.vi"("error in (no error)"=w467, "FPGA VI Reference Out"=w465) -> ("error out"=w466:errorcluster)  [unwired: 9 in]
    n185 = shared-variable "NI-cRIO-9048-02018485\\Host-Target shared variables.lvlib\\FPGA Routine 1 Pulsing"(error in=w466) -> (w469:T3, error out=w472:errorcluster)
    n186 = Unbundle By Name(w469) -> ("Pulsing"=w470:bool)
    n187 = feedback-in #1(w470) -> ()
    n188 = feedback #1(FALSE ("Start Pulsing")) -> (w474:bool)
    n189 = Not Equal?(x=w474, y=w470) -> (x != y?=w473:bool)
    n190 = case shown="True" w473 {
      tunnel: w472 -> [w480 w484]
      tunnel: [w480 w482] -> w471
      tunnel: w470 -> [_ w485]
      tunnel: w469 -> [_ w483]
      tunnel: w465 -> [_ w481]
      frame False {
      }
      frame True {
        n191 = case shown="True" w485 {
          tunnel: w484 -> [w489 w501]
          tunnel: w483 -> [_ w500]
          tunnel: [w488 w493] -> w482
          tunnel: w481 -> [w487 w492]
          frame False {
            n192 = xnode "Read/Write Control"("FPGA VI Reference In"=w487, "error in"=w489, "Stop Routine"=TRUE) -> ("error out"=w488:errorcluster)  [unwired: 1 out]
          }
          frame True {
            n193 = Unbundle By Name(w500) -> ("Pulse Period (uS)"=w491:u32, "Pulse duration (uS)"=w490:u32)
            n194 = xnode "Read/Write Control"("FPGA VI Reference In"=w492, "error in"=w501, "Pulse Period"=w491, "Pulse Width"=w490) -> ("FPGA VI Reference Out"=w498:refnum<k20>, "error out"=w499:errorcluster)
            n195 = xnode "Invoke Method"("FPGA VI Reference In"=w498, "error in"=w499, "IRQ Number(s)"=8) -> ("FPGA VI Reference Out"=w496:refnum<k20>, "error out"=w495:errorcluster, "IRQ(s) Asserted"=w494:i32)  [unwired: 1 in, 1 out]
            n196 = xnode "Invoke Method"("FPGA VI Reference In"=w496, "error in"=w495, "IRQ Number(s)"=w494) -> ("error out"=w493:errorcluster)  [unwired: 1 out]
          }
        }
      }
    }
  }
  n197 = Merge Errors(w4, w8, w12, w11, w3) -> (w10:errorcluster)
  n198 = call "Shut Down.vi"("error in (no error)"=w10, "FPGA VI Reference Out"=w1) -> ()  [unwired: 10 in]
